vi "serialize.vi"(8 "error in":errorcluster, 11 "Results":T1[](array[typedef])) -> (0 "error out":errorcluster, 3 "serialized results":string)   [LabVIEW 2014]
uses:
  xml format - file.ctl
  xml format - error.ctl
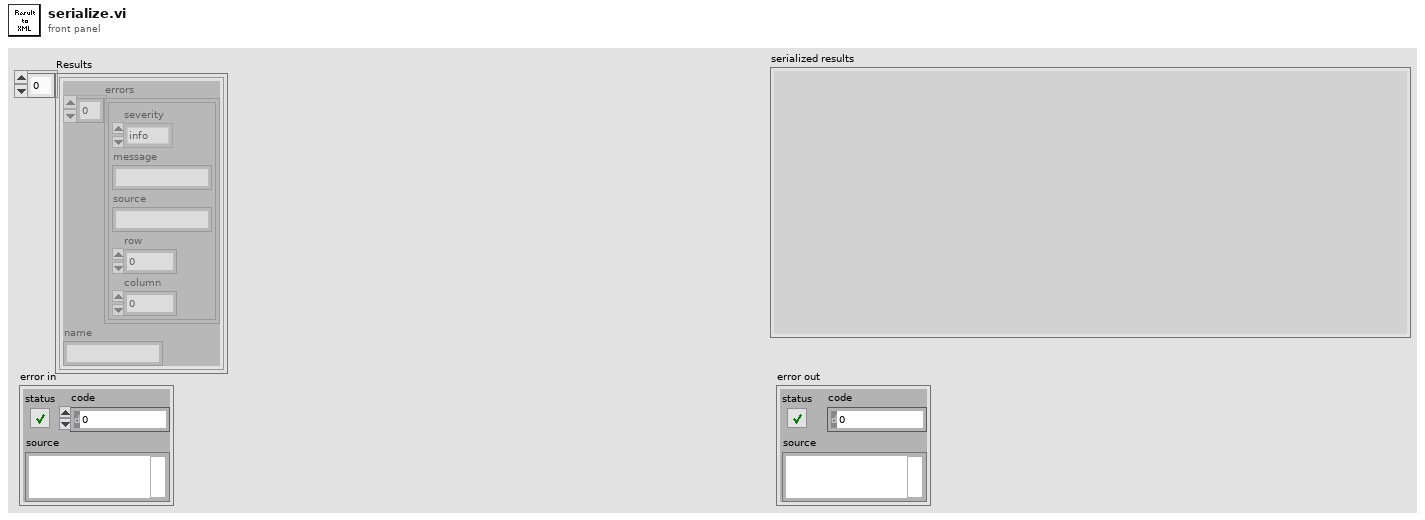
[diagram p1: front panel]
types:
  T1 = typedef "xml format - file.ctl" = cluster{"errors":T2[], "name":string}
  T2 = typedef "xml format - error.ctl" = cluster{"severity":enum16{"info", "warning", "error"}, "message":string, "source":string, "row":i32, "column":i32}
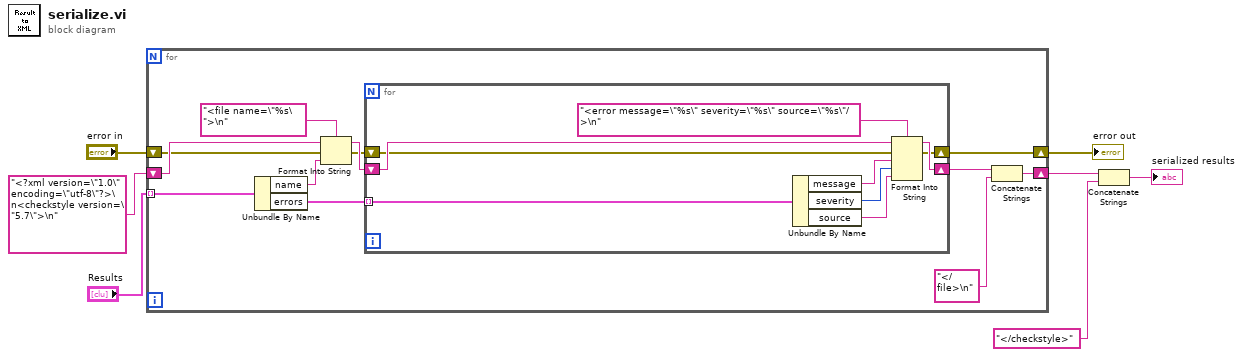
[diagram p0: block diagram]
diagram:
  n1 = for {
    tunnel: "Results" -> [w19] mode=indexing
    shift-right: [w13] -> w1
    shift-left: "error in" -> [w11]
    shift-right: [w8] -> w5
    shift-left: "<?xml version=\"1.0\" encoding=\"utf-8\"?>\n<checkstyle version=\"5.7\">\n" -> [w12]
    n2 = Unbundle By Name(w19) -> ("name"=w17:string, "errors"=w16:T2[])
    n3 = Format Into String(format string="<file name=\"%s\">\n", initial string=w12, error in=w11, w17) -> (resulting string=w15:string, error out=w14:errorcluster)
    n4 = for {
      tunnel: w16 -> [w28] mode=indexing
      shift-right: [w26] -> w10
      shift-left: w15 -> [w27]
      shift-right: [w24] -> w13
      shift-left: w14 -> [w25]
      n5 = Unbundle By Name(w28) -> ("message"=w22:string, "severity"=w21:enum16{"info", "warning", "error"}, "source"=w20:string)
      n6 = Format Into String(format string="<error message=\"%s\" severity=\"%s\" source=\"%s\"/>\n", initial string=w27, error in=w25, w22, w21, w20) -> (resulting string=w26:string, error out=w24:errorcluster)
    }
    n7 = Concatenate Strings(w10, "</file>\n" ("string")) -> (w8:string)
  }
  "error out" <- w1
  n8 = Concatenate Strings(w5, "</checkstyle>") -> (→"serialized results":string)
